vi "shipingWithSubLot.vi"(11 "template (empty)":path=path "O:/Monitor/回貨明細_1106.xls") -> (0 "error out":errorcluster, 3 "report out":refnum<class "NI_report.lvclass">)   [LabVIEW 2012]
uses:
  <vilib>/Utility/NIReport.llb/NI_report.lvclass
  Global1.vi
  <vilib>/addons/database/Connection.llb/DB Tools Open Connec (Path).vi
  <vilib>/addons/_office/excel.llb/Excel Get Data (str).vi
  <vilib>/Utility/NIReport.llb/Excel/NI_Excel.lvclass
  <vilib>/addons/_office/NI_ReportGenerationToolkit.lvlib
  <vilib>/addons/database/NI_Database_API.lvlib
panel:
  out "Numeric":i32
  in  "start (0, 0)":cluster{"start row":i32, "start column":i32}
  out "Numeric 2":i32
  out "row":i32
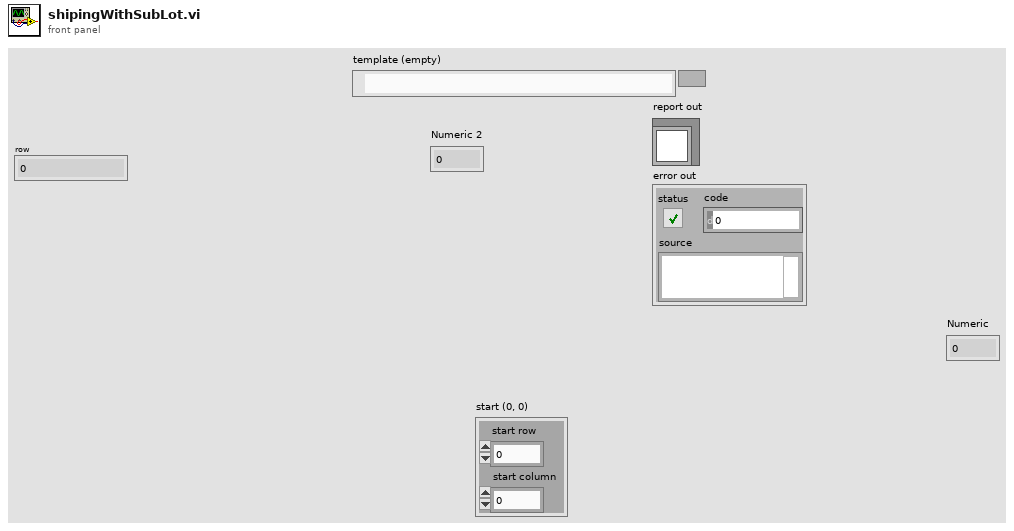
[diagram p1: front panel]
types:
  T1 = enum16{"Standard Report", "HTML", "Word", "Excel"}
  T2 = typedef "NI_Database_API.lvlib/Conn ObjectReference.ctl" = refnum<k1>
  T3 = cluster{"on/off":bool, "weight":i32, "color":u32}
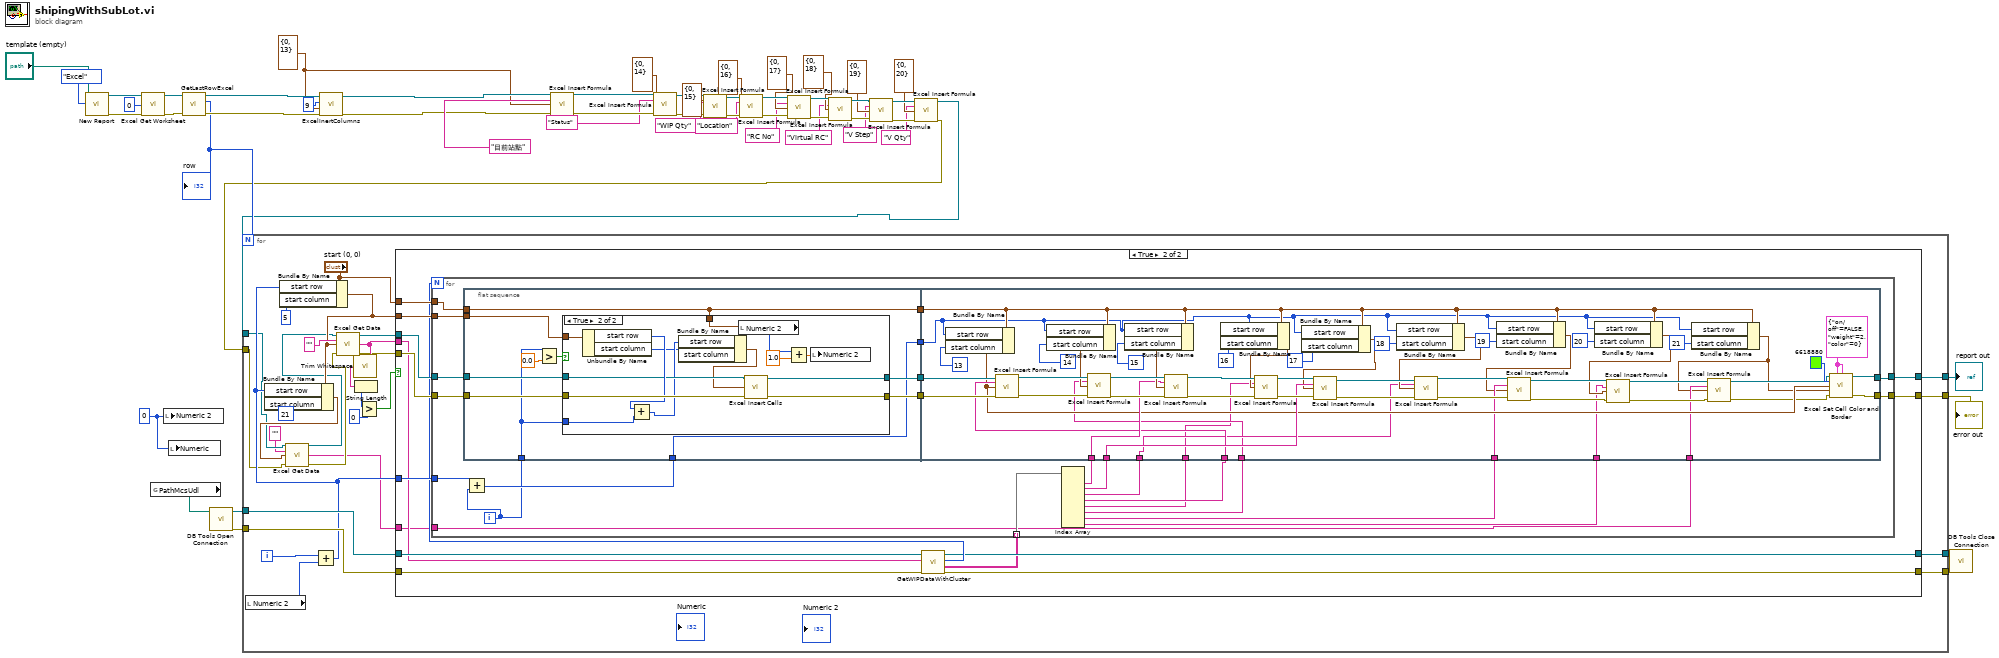
[diagram p0: block diagram]
diagram:
  w26 = 0
  w30 = cluster{"row":i32, "column":i32} {"row"=0, "column"=13} ("start (0, 0)")
  n1 = call <vilib>:"New Report.vi"("report type"=T1."Excel" ("Report Type"), "template (empty)"="template (empty)") -> ("report out"=w52:refnum<class "NI_report.lvclass">, "error out"=w51:errorcluster)  [unwired: 12 in]
  n2 = call <vilib>:"Excel Get Worksheet.vi"("report in"=w52, "worksheet index (0)"=0, "error in (no error)"=w51) -> ("report out"=w43:refnum<class "NI_report.lvclass">, "error out"=w42:errorcluster)  [unwired: 11 in]
  n3 = global read "Global1.vi" "PathMcsUdl"() -> (w21:path)
  n4 = local write "Numeric 2"(w26) -> ()
  n5 = local write "Numeric"(w26) -> ()
  n6 = call "GetLastRowExcel.vi"("error in (no error)"=w42, "report in"=w43) -> ("error out"=w34:errorcluster, "row"=w27:i32, "report out"=w35:refnum<class "NI_report.lvclass">)  [unwired: 7 in]
  "row" <- w27
  n7 = call-poly <vilib>:"DB Tools Open Connection.vi"("connection information"=w21) -> ("error out"=w24:errorcluster, "connection reference"=w25:T2)  [unwired: 7 in]
  n8 = call "ExcelInertColumns.vi"("error in (no error)"=w34, "start (0, 0)"=w30, "Numeric"=9, "report in"=w35) -> ("error out"=w31:errorcluster, "report out"=w32:refnum<class "NI_report.lvclass">)  [unwired: 6 in]
  n9 = call <vilib>:"Excel Insert Formula.vi"("report in"=w32, "formula"="目前站點", "start (0, 0)"=w30, "error in (no error)"=w31) -> ("report out"=w50:refnum<class "NI_report.lvclass">, "error out"=w48:errorcluster)  [unwired: 10 in]
  n10 = call <vilib>:"Excel Insert Formula.vi"("report in"=w50, "formula"="Status", "start (0, 0)"=cluster{"row":i32, "column":i32} {"row"=0, "column"=14}, "error in (no error)"=w48) -> ("report out"=w49:refnum<class "NI_report.lvclass">, "error out"=w47:errorcluster)  [unwired: 10 in]
  n11 = call <vilib>:"Excel Insert Formula.vi"("report in"=w49, "formula"="WIP Qty", "start (0, 0)"=cluster{"row":i32, "column":i32} {"row"=0, "column"=15}, "error in (no error)"=w47) -> ("report out"=w41:refnum<class "NI_report.lvclass">, "error out"=w40:errorcluster)  [unwired: 10 in]
  n12 = call <vilib>:"Excel Insert Formula.vi"("report in"=w41, "formula"="Location", "start (0, 0)"=cluster{"row":i32, "column":i32} {"row"=0, "column"=16}, "error in (no error)"=w40) -> ("report out"=w20:refnum<class "NI_report.lvclass">, "error out"=w19:errorcluster)  [unwired: 10 in]
  n13 = call <vilib>:"Excel Insert Formula.vi"("report in"=w20, "formula"="RC No", "start (0, 0)"=cluster{"row":i32, "column":i32} {"row"=0, "column"=17}, "error in (no error)"=w19) -> ("report out"=w14:refnum<class "NI_report.lvclass">, "error out"=w13:errorcluster)  [unwired: 10 in]
  n14 = call <vilib>:"Excel Insert Formula.vi"("report in"=w14, "formula"="Virtual RC", "start (0, 0)"=cluster{"row":i32, "column":i32} {"row"=0, "column"=18}, "error in (no error)"=w13) -> ("report out"=w10:refnum<class "NI_report.lvclass">, "error out"=w7:errorcluster)  [unwired: 10 in]
  n15 = call <vilib>:"Excel Insert Formula.vi"("report in"=w10, "formula"="V Step", "start (0, 0)"=cluster{"row":i32, "column":i32} {"row"=0, "column"=19}, "error in (no error)"=w7) -> ("report out"=w9:refnum<class "NI_report.lvclass">, "error out"=w6:errorcluster)  [unwired: 10 in]
  n16 = call <vilib>:"Excel Insert Formula.vi"("report in"=w9, "formula"="V Qty", "start (0, 0)"=cluster{"row":i32, "column":i32} {"row"=0, "column"=20}, "error in (no error)"=w6) -> ("report out"=w8:refnum<class "NI_report.lvclass">, "error out"=w5:errorcluster)  [unwired: 10 in]
  n17 = for {
    N: w27 -> [_]
    tunnel: w8 -> [w58]
    tunnel: w5 -> [w59]
    tunnel: [w71] -> w16
    tunnel: [w70] -> w15
    tunnel: w25 -> [w67]
    tunnel: w24 -> [w66]
    tunnel: [w65] -> w23
    tunnel: [w64] -> w22
    i -> [w69]
    n18 = local read "Numeric 2"() -> (w68:i32)
    n19 = Add(x=w69, y=w68) -> (x+y=w62:i32)
    n20 = Bundle By Name(cluster="start (0, 0)", "start row"=w62, "start column"=5) -> (w60:cluster{"start row":i32, "start column":i32})
    n21 = Bundle By Name(cluster=w60, "start row"=w62, "start column"=21) -> (w61:cluster{"start row":i32, "start column":i32})
    n22 = call-poly <vilib>:"Excel Get Data.vi"("report in"=w58, "data type"="", "start (0, 0)"=w61, "error in (no error)"=w59) -> ("report out"=w56:refnum<class "NI_report.lvclass">, "data"=w54:string, "error out"=w55:errorcluster)  [unwired: 9 in]
    n23 = call-poly <vilib>:"Excel Get Data.vi"("report in"=w56, "data type"="", "start (0, 0)"=w60, "error in (no error)"=w55) -> ("report out"=w73:refnum<class "NI_report.lvclass">, "data"=w75:string, "error out"=w72:errorcluster)  [unwired: 9 in]
    n24 = call <vilib>:"Trim Whitespace.vi"("string"=w75) -> ("trimmed string"=w78:string)  [unwired: 1 in]
    n25 = String Length(string=w78) -> (length=w77:i32)
    n26 = Greater?(x=w77, y=0) -> (0:w76:bool)
    n27 = case shown="True" w76 {
      tunnel: w75 -> [_ w91]
      tunnel: "start (0, 0)" -> [_ w100]
      tunnel: w73 -> [w85 w99]
      tunnel: w72 -> [w84 w98]
      tunnel: [w85 w97] -> w71
      tunnel: [w84 w96] -> w70
      tunnel: w62 -> [_ w95]
      tunnel: w60 -> [_ w94]
      tunnel: w67 -> [w83 w93]
      tunnel: w66 -> [w82 w92]
      tunnel: [w83 w89] -> w65
      tunnel: [w82 w88] -> w64
      tunnel: w54 -> [_ w86]
      frame False {
      }
      frame True {
        n28 = call "GetWIPDataWithCluster.vi"("error in"=w92, "Lotno"=w91, "connection reference"=w93) -> ("error out"=w88:errorcluster, "output array"=w87:string[][], "data"=w90:i32, "connection reference 2"=w89:T2)  [unwired: 5 in]
        n29 = for {
          N: w90 -> [_]
          tunnel: w99 -> [w123]
          tunnel: [w122] -> w97
          tunnel: w100 -> [w121]
          tunnel: w98 -> [w120]
          tunnel: [w119] -> w96
          tunnel: w95 -> [w118]
          tunnel: w94 -> [w112]
          tunnel: w87 -> [w111] mode=indexing
          tunnel: w86 -> [w103]
          i -> [w110]
          n30 = flat-sequence {
            tunnel: w123 -> [w128]
            tunnel: w121 -> [w125]
            tunnel: [w125] -> w116
            tunnel: w120 -> [w127]
            tunnel: w117 -> [w129]
            tunnel: [w129] -> w115
            tunnel: [w131] -> w114
            tunnel: [w130] -> w113
            tunnel: w110 -> [w124]
            tunnel: w112 -> [w126]
            tunnel: w116 -> [w158]
            tunnel: w115 -> [w157]
            tunnel: [w181] -> w122
            tunnel: w114 -> [w189]
            tunnel: [w180] -> w119
            tunnel: w113 -> [w188]
            tunnel: w109 -> [w184]
            tunnel: w108 -> [w183]
            tunnel: w107 -> [w171]
            tunnel: w106 -> [w182]
            tunnel: w105 -> [w150]
            tunnel: w104 -> [w151]
            tunnel: w102 -> [w168]
            tunnel: w103 -> [w154]
            tunnel: w101 -> [w153]
            frame #0 {
              n31 = Greater?(x=w124, y=0.0) -> (0:w132:bool)
              n32 = case shown="True" w132 {
                tunnel: [w135 w149] -> w131
                tunnel: [w134 w148] -> w130
                tunnel: w128 -> [w135 w141]
                tunnel: w127 -> [w134 w144]
                tunnel: w126 -> [_ w143]
                tunnel: w125 -> [_ w140]
                tunnel: w124 -> [_ w136]
                frame False {
                }
                frame True {
                  n33 = Unbundle By Name(w143) -> ("start row"=w142:i32, "start column"=w138:i32)
                  n34 = Add(x=w142, y=w136) -> (x+y=w139:i32)
                  n35 = Bundle By Name(cluster=w140, "start row"=w139, "start column"=w138) -> (w137:cluster{"start row":i32, "start column":i32})
                  n36 = local read "Numeric 2"() -> (w147:i32)
                  n37 = call <vilib>:"Excel Insert Cells.vi"("report in"=w141, "start (0, 0)"=w137, "error in (no error)"=w144) -> ("report out"=w149:refnum<class "NI_report.lvclass">, "error out"=w148:errorcluster)  [unwired: 11 in]
                  n38 = Add(x=w147, y=1.0) -> (x+y=w145:dbl)
                  n39 = local write "Numeric 2"(w145) -> ()
                }
              }
            }
            frame #1 {
              w176 = T3 {"on/off"=FALSE, "weight"=2, "color"=0} ("inside border")
              n40 = Bundle By Name(cluster=w158, "start row"=w157, "start column"=13) -> (w178:cluster{"start row":i32, "start column":i32})
              n41 = call <vilib>:"Excel Insert Formula.vi"("report in"=w189, "formula"=w182, "start (0, 0)"=w178, "error in (no error)"=w188) -> ("report out"=w199:refnum<class "NI_report.lvclass">, "error out"=w196:errorcluster)  [unwired: 10 in]
              n42 = Bundle By Name(cluster=w158, "start row"=w157, "start column"=14) -> (w194:cluster{"start row":i32, "start column":i32})
              n43 = call <vilib>:"Excel Insert Formula.vi"("report in"=w199, "formula"=w151, "start (0, 0)"=w194, "error in (no error)"=w196) -> ("report out"=w198:refnum<class "NI_report.lvclass">, "error out"=w197:errorcluster)  [unwired: 10 in]
              n44 = Bundle By Name(cluster=w158, "start row"=w157, "start column"=15) -> (w195:cluster{"start row":i32, "start column":i32})
              n45 = call <vilib>:"Excel Insert Formula.vi"("report in"=w198, "formula"=w184, "start (0, 0)"=w195, "error in (no error)"=w197) -> ("report out"=w192:refnum<class "NI_report.lvclass">, "error out"=w191:errorcluster)  [unwired: 10 in]
              n46 = Bundle By Name(cluster=w158, "start row"=w157, "start column"=16) -> (w190:cluster{"start row":i32, "start column":i32})
              n47 = call <vilib>:"Excel Insert Formula.vi"("report in"=w192, "formula"=w150, "start (0, 0)"=w190, "error in (no error)"=w191) -> ("report out"=w186:refnum<class "NI_report.lvclass">, "error out"=w185:errorcluster)  [unwired: 10 in]
              n48 = Bundle By Name(cluster=w158, "start row"=w157, "start column"=17) -> (w177:cluster{"start row":i32, "start column":i32})
              n49 = call <vilib>:"Excel Insert Formula.vi"("report in"=w186, "formula"=w183, "start (0, 0)"=w177, "error in (no error)"=w185) -> ("report out"=w174:refnum<class "NI_report.lvclass">, "error out"=w173:errorcluster)  [unwired: 10 in]
              n50 = Bundle By Name(cluster=w158, "start row"=w157, "start column"=18) -> (w172:cluster{"start row":i32, "start column":i32})
              n51 = call <vilib>:"Excel Insert Formula.vi"("report in"=w174, "formula"=w171, "start (0, 0)"=w172, "error in (no error)"=w173) -> ("report out"=w167:refnum<class "NI_report.lvclass">, "error out"=w170:errorcluster)  [unwired: 10 in]
              n52 = Bundle By Name(cluster=w158, "start row"=w157, "start column"=19) -> (w166:cluster{"start row":i32, "start column":i32})
              n53 = call <vilib>:"Excel Insert Formula.vi"("report in"=w167, "formula"=w168, "start (0, 0)"=w166, "error in (no error)"=w170) -> ("report out"=w160:refnum<class "NI_report.lvclass">, "error out"=w163:errorcluster)  [unwired: 10 in]
              n54 = Bundle By Name(cluster=w158, "start row"=w157, "start column"=20) -> (w159:cluster{"start row":i32, "start column":i32})
              n55 = call <vilib>:"Excel Insert Formula.vi"("report in"=w160, "formula"=w153, "start (0, 0)"=w159, "error in (no error)"=w163) -> ("report out"=w165:refnum<class "NI_report.lvclass">, "error out"=w162:errorcluster)  [unwired: 10 in]
              n56 = Bundle By Name(cluster=w158, "start row"=w157, "start column"=21) -> (w152:cluster{"start row":i32, "start column":i32})
              n57 = call <vilib>:"Excel Insert Formula.vi"("report in"=w165, "formula"=w154, "start (0, 0)"=w152, "error in (no error)"=w162) -> ("report out"=w164:refnum<class "NI_report.lvclass">, "error out"=w161:errorcluster)  [unwired: 10 in]
              n58 = call <vilib>:"Excel Set Cell Color and Border.vi"("report in"=w164, "inside border"=w176, "outside border"=w176, "background color (w)"=u32 6618880, "start (-1, -1)"=w178, "end (-1, -1)"=w152, "error in (no error)"=w161) -> ("report out"=w181:refnum<class "NI_report.lvclass">, "error out"=w180:errorcluster)  [unwired: 7 in]
            }
          }
          n59 = Add(x=w118, y=w110) -> (x+y=w117:i32)
          n60 = Index Array(array=w111) -> (element #1=w109:string, element #2=w108:string, element #3=w107:string, element #4=w106:string, element #5=w105:string, element #6=w104:string, element #7=w102:string, element #8=w101:string)  [unwired: 8 in]
        }
      }
    }
  }
  "report out" <- w16
  "error out" <- w15
  n61 = call <vilib>:"DB Tools Close Connection.vi"("error in (no error)"=w22, "connection reference"=w23) -> ()  [unwired: 5 in, 1 out]
